vi "Untitled 10.vi"() -> ()   [LabVIEW 2013]
panel:
  out "Real 3":dbl
  out "Real 2":dbl
  out "Real":dbl
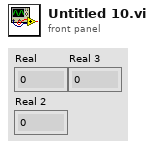
[diagram p1: front panel]
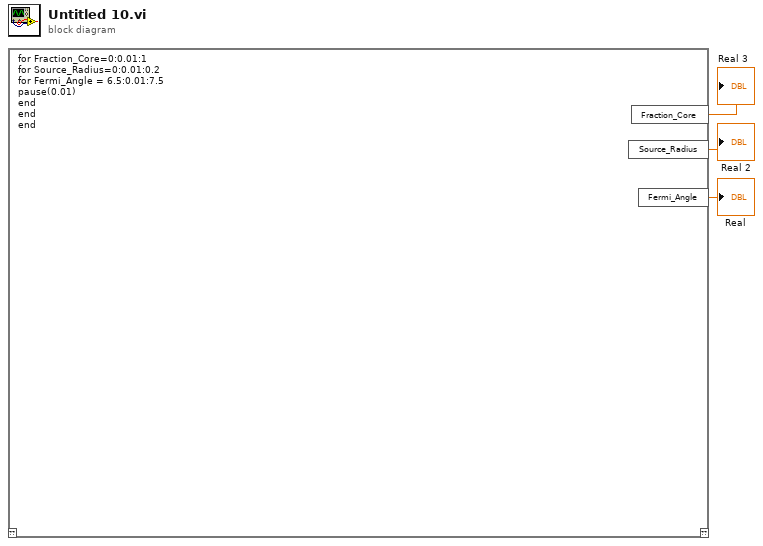
[diagram p0: block diagram]
diagram:
  n1 = script code="for Fraction_Core=0:0.01:1\nfor Source_Radius=0:0.01:0.2\nfor Fermi_Angle = 6.5:0.01:7.5\npause(0.01)\nend\nend\nend"() -> ("Fraction_Core"=→"Real 3":dbl, "Source_Radius"=→"Real 2":dbl, "Fermi_Angle"=→"Real":dbl)  [unwired: 1 in, 1 out]
